vi "UpdateTECEn.vi"(7 "LabVIEW Web Service Request":refnum<class "Web Request.lvclass">, 11 "TECEnByte":u8) -> ()   [LabVIEW 2014]
uses:
  Controller/Controller.lvclass
  Controller/Controls/Enqueuer Enum.ctl
  <vilib>/wsapi/Web Request.lvclass
  Instr Actor/Messages/Set TEC SP MSG/Set TEC Enable MSG.lvclass
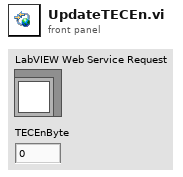
[diagram p1: front panel]
types:
  T1 = typedef "Controller.lvlib/Controller.lvclass/Enqueuer Enum.ctl" = enum8{"PAS", "CRDS", "File", "O3Lamp"}
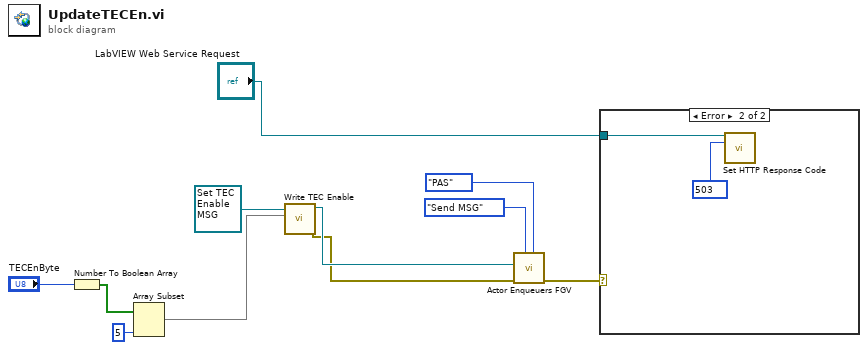
[diagram p0: block diagram]
diagram:
  n1 = Number To Boolean Array(number="TECEnByte") -> (Boolean array=w7:bool[])
  n2 = Array Subset(array=w7, length=5) -> (w3:bool[])  [unwired: 1 in]
  n3 = call "Write TEC Enable.vi"("TEC Enable"=w3, "Set TEC Enable MSG in"=refnum<class "Set TEC Enable MSG.lvclass"> refnum ("Instrument Lib:Set TEC Enable MSG.lvclass")) -> ("error out"=w1:errorcluster, "Set TEC Enable MSG out"=w2:refnum<class "Set TEC Enable MSG.lvclass">)  [unwired: 8 in]
  n4 = call "Actor Enqueuers FGV.vi"("Enqueuer"=Enqueuer_Enum."PAS", "State"=enum16{"Store", "Send MSG"}."Send MSG", "error in"=w1, "MSG"=w2) -> ("error out"=w9:errorcluster)  [unwired: 7 in]
  n5 = case shown="Error" w9 {
    tunnel: "LabVIEW Web Service Request" -> [_ w12]
    frame No Error {
    }
    frame Error {
      w13 = 503 items=["100"=100, "101"=101, "200"=200, "201"=201, "202"=202, "203"=203, "204"=204, "205"=205, "206"=206, "300"=300, "301"=301, "302"=302, "303"=303, "304"=304, "305"=305, "306"=306, "307"=307, "400"=400, "401"=401, "402"=402, "403"=403, "404"=404, "405"=405, "406"=406, "407"=407, "408"=408, "409"=409, "410"=410, "411"=411, "412"=412, "413"=413, "414"=414, "415"=415, "416"=416, "417"=417, "500"=500, "501"=501, "502"=502, "503"=503, "504"=504, "505"=505] ("response code (200)")
      n6 = call <vilib>:"Set HTTP Response Code.vi"("LabVIEW Web Service Request"=w12, "response code (200)"=w13) -> ()  [unwired: 12 in, 2 out]
    }
  }
